vi "AD.vi"() -> ()   [LabVIEW 2018]
uses:
  work2020/SARController/SAR-Controller/main/PCI8552B_32.dll
panel:
  out "Data":dbl[][](array[numeric])
  out "波形图":dbl[][](graph)
  out "待读取数据长度":i32
  in  "STOP":bool
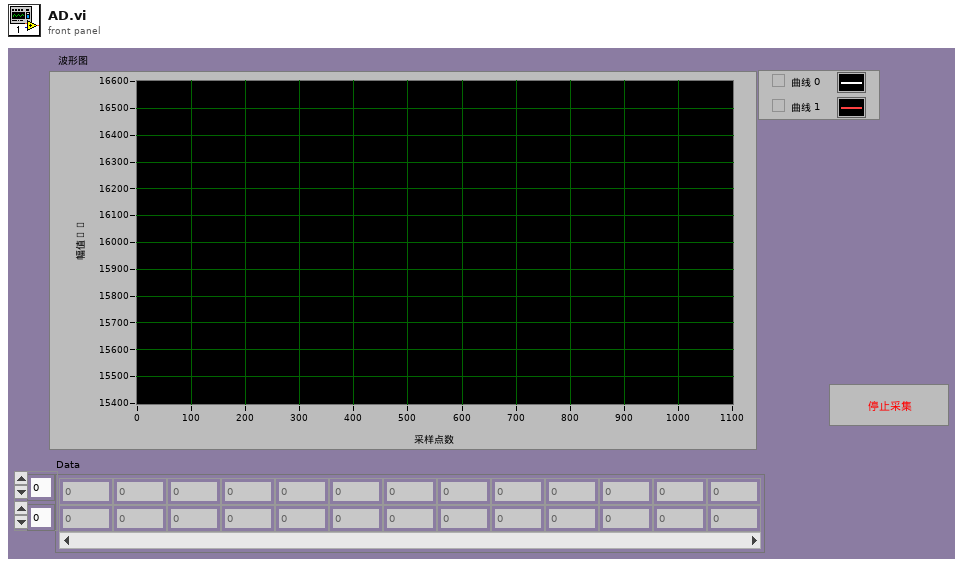
[diagram p1: front panel]
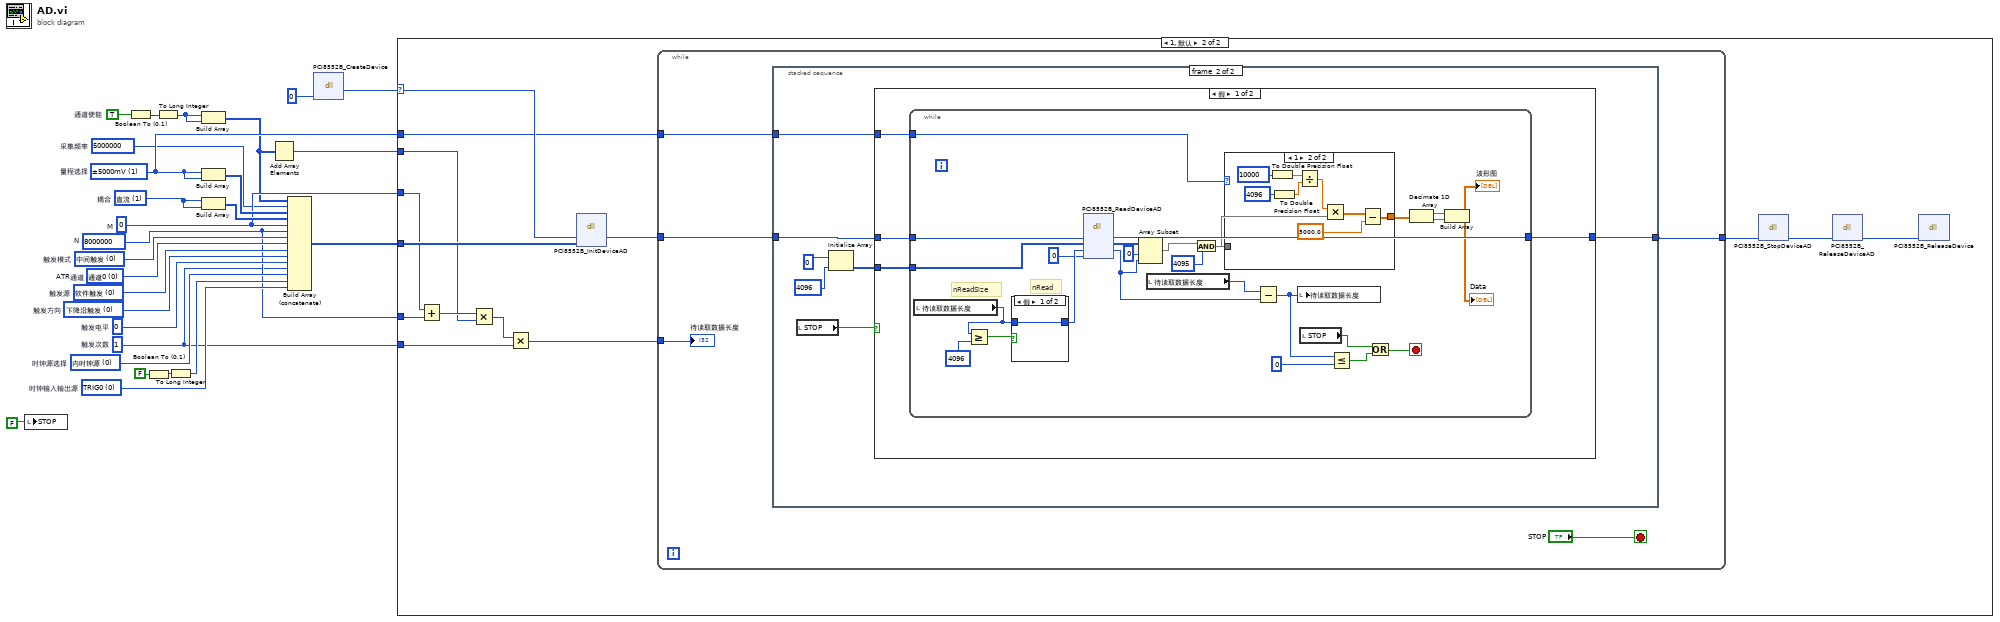
[diagram p0: block diagram]
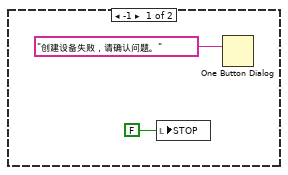
[diagram p2: hidden frame]
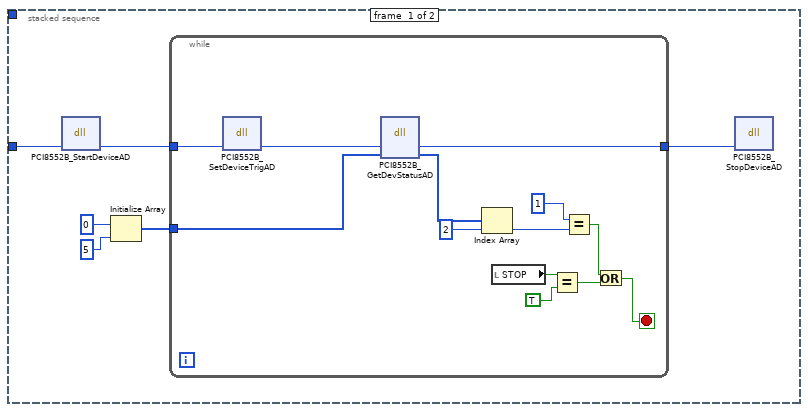
[diagram p3: hidden frame]
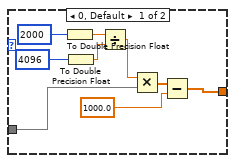
[diagram p4: hidden frame]
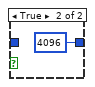
[diagram p5: hidden frame]
diagram:
  w6 = 8000000  # N
  w7 = 0  # M
  w8 = 1 items=["交流", "直流"]  # 耦合
  w3 = 1 items=["±1000mV", "±5000mV"]  # 量程选择
  w10 = TRUE  # 通道使能
  w1 = 5000000  # 采集频率
  w16 = 0 items=["中间触发", "后触发", "预触发", "硬件延时触发"]  # 触发模式
  w13 = 0 items=["通道0", "通道1"]  # ATR通道
  w25 = 0 items=["软件触发", "DTR作为触发源", "ATR作为触发源", "Trigger信号触发"]  # 触发源
  w24 = 0 items=["下降沿触发", "上升沿触发", "上下边沿均触发", ""]  # 触发方向
  w23 = 0  # 触发电平
  w4 = 1  # 触发次数
  w21 = 0 items=["TRIG0", "TRIG1", "TRIG2", "TRIG3"]  # 时钟输入输出源
  w22 = 0 items=["内时钟源", "主卡10M时钟源", "外部时钟"]  # 时钟源选择
  n1 = local write "STOP"(FALSE) -> ()
  n2 = Boolean To (0,1)(Boolean=w10) -> (0, 1=w18:i16)
  n3 = Boolean To (0,1)(Boolean=FALSE ("主设备使能")) -> (0, 1=w19:i16)
  n4 = To Long Integer(number=w18) -> (32bit integer=w9:i32)
  n5 = To Long Integer(number=w19) -> (32bit integer=w20:i32)
  n6 = Build Array(w9, w9) -> (w2:i32[])
  n7 = Build Array(w3, w3) -> (w15:i32[])
  n8 = Build Array(w8, w8) -> (w26:i32[])
  n9 = Add Array Elements(numeric array=w2) -> (sum=w5:i32)
  n10 = Build Array (concatenate)(w2, w1, w15, w26, w7, w6, w16, w13, w25, w24, w23, w4, w22, w20, w21) -> (w17:i32[])
  n11 = dll-call lib="PTH2…abs E\nPersonal Fileç ”ç©¶ç”Ÿå­¦ä¹ 202002-202007ç ”ä¸€ä¸‹å­¦æœŸwork2020\nSARControllerSAR-ControllermainPCI8552B_32.DLL" fn="PCI8552B_CreateDevice" label="CreateDevice"("DeviceLgcID"=0) -> ("返回类型"=w11:i32)  [unwired: 4 in, 2 out]
  n12 = case shown="1, 默认" w11 {
    selector: w11 -> [_ w31]
    tunnel: w17 -> [_ w41]
    tunnel: w7 -> [_ w40]
    tunnel: w6 -> [_ w39]
    tunnel: w5 -> [_ w37]
    tunnel: w4 -> [_ w35]
    tunnel: w3 -> [_ w30]
    frame -1 {
      n13 = local write "STOP"(FALSE) -> ()
      n14 = One Button Dialog(message="创建设备失败，请确认问题。") -> ()  [unwired: 1 in, 1 out]
    }
    frame 1, Default {
      n15 = Add(x=w40, y=w39) -> (x+y=w38:i32)
      n16 = Multiply(x=w38, y=w37) -> (x*y=w36:i32)
      n17 = Multiply(x=w36, y=w35) -> (x*y=w34:i32)
      n18 = dll-call lib="PTH2…abs E\nPersonal Fileç ”ç©¶ç”Ÿå­¦ä¹ 202002-202007ç ”ä¸€ä¸‹å­¦æœŸwork2020\nSARControllerSAR-ControllermainPCI8552B_32.DLL" fn="PCI8552B_InitDeviceAD" label="InitDeviceAD"("hDevice"=w31, "pADPara"=w41) -> ("hDevice"=w42:i32)  [unwired: 5 in, 2 out]
      n19 = while {
        tunnel: [w48] -> w43
        tunnel: w42 -> [w46]
        tunnel: w34 -> [w47]
        tunnel: w30 -> [w44]
        stop <- "STOP" stop-if-true
        n20 = stacked-sequence {
          tunnel: w46 -> [w50 w69]
          tunnel: [_ w74] -> w48
          tunnel: w44 -> [_ w68]
          frame #0 {
            n21 = dll-call lib="PTH2…abs E\nPersonal Fileç ”ç©¶ç”Ÿå­¦ä¹ 202002-202007ç ”ä¸€ä¸‹å­¦æœŸwork2020\nSARControllerSAR-ControllermainPCI8552B_32.DLL" fn="PCI8552B_StartDeviceAD" label="StartDeviceAD"("hDevice"=w50) -> ("hDevice"=w49:i32)  [unwired: 4 in, 2 out]
            n22 = Initialize Array(0, 5) -> (w54:i32[])
            n23 = while {
              tunnel: w49 -> [w57]
              tunnel: w54 -> [w67]
              tunnel: [w55] -> w51
              stop <- w58 stop-if-true
              n24 = dll-call lib="PTH2…abs E\nPersonal Fileç ”ç©¶ç”Ÿå­¦ä¹ 202002-202007ç ”ä¸€ä¸‹å­¦æœŸwork2020\nSARControllerSAR-ControllermainPCI8552B_32.DLL" fn="PCI8552B_SetDeviceTrigAD" label="SetDeviceTrigAD"("hDevice"=w57) -> ("hDevice"=w56:i32)  [unwired: 4 in, 2 out]
              n25 = dll-call lib="PTH2…abs E\nPersonal Fileç ”ç©¶ç”Ÿå­¦ä¹ 202002-202007ç ”ä¸€ä¸‹å­¦æœŸwork2020\nSARControllerSAR-ControllermainPCI8552B_32.DLL" fn="PCI8552B_GetDevStatusAD" label="GetDevStatusAD"("hDevice"=w56, "ADStatus"=w67) -> ("hDevice"=w55:i32, "ADStatus"=w63:i32[])  [unwired: 4 in, 2 out]
              n26 = Index Array(array=w63, index=2) -> (element=w65:i32)
              n27 = local read "STOP"() -> (w62:bool)
              n28 = Equal?(x=w62, y=TRUE) -> (x = y?=w59:bool)
              n29 = Equal?(x=1, y=w65) -> (x = y?=w60:bool)
              n30 = Or(x=w60, y=w59) -> (x .or. y?=w58:bool)
            }
            n31 = dll-call lib="PTH2…abs E\nPersonal Fileç ”ç©¶ç”Ÿå­¦ä¹ 202002-202007ç ”ä¸€ä¸‹å­¦æœŸwork2020\nSARControllerSAR-ControllermainPCI8552B_32.DLL" fn="PCI8552B_StopDeviceAD" label="StopDeviceAD"("hDevice"=w51) -> ()  [unwired: 5 in, 2 out]
          }
          frame #1 {
            n32 = local read "STOP"() -> (w70:bool)
            n33 = Initialize Array(u16 0 ("y"), 4096 ("y")) -> (w71:u16[])
            n34 = case shown="假" w70 {
              tunnel: w69 -> [w78 w124]
              tunnel: [w77 w124] -> w74
              tunnel: w71 -> [w76 _]
              tunnel: w68 -> [w75 _]
              frame False {
                n35 = while {
                  tunnel: w78 -> [w103]
                  tunnel: [w102] -> w77
                  tunnel: w76 -> [w101]
                  tunnel: w75 -> [w88]
                  stop <- w96 stop-if-true
                  # "nReadSize"
                  # "nRead"
                  n36 = local read "待读取数据长度"() -> (w95:i32)
                  n37 = Greater Or Equal?(x=w95, y=4096 ("millisecond multiple")) -> (x >= y?=w99:bool)
                  n38 = case shown="假" w99 {
                    tunnel: [w122 4096 ("millisecond multiple")] -> w92
                    tunnel: w95 -> [w122 _]
                    frame False {
                    }
                    frame True {
                    }
                  }
                  n39 = dll-call lib="PTH2…abs E\nPersonal Fileç ”ç©¶ç”Ÿå­¦ä¹ 202002-202007ç ”ä¸€ä¸‹å­¦æœŸwork2020\nSARControllerSAR-ControllermainPCI8552B_32.DLL" fn="PCI8552B_ReadDeviceAD" label="ReadDeviceAD"("hDevice"=w103, "pADBuffer"=w101, "nReadSizeWords"=w92, "nRetSizeWords"=0) -> ("hDevice"=w102:i32, "pADBuffer"=w85:u16[], "nReadSizeWords"=w82:u32)  [unwired: 5 in, 2 out]
                  n40 = Array Subset(array=w85, index=0 ("索引"), length=w82) -> (w84:u16[])
                  n41 = local read "待读取数据长度"() -> (w94:i32)
                  n42 = And(x=w84, y=u16 4095) -> (x .and. y?=w89:u16[])
                  n43 = case shown="1" w88 {
                    tunnel: w89 -> [w111 w116]
                    tunnel: [w104 w115] -> w87
                    frame 0, Default {
                      n44 = To Double Precision Float(number=2000 ("x")) -> (double precision float=w107:dbl)
                      n45 = To Double Precision Float(number=4096) -> (double precision float=w106:dbl)
                      n46 = Divide(x=w107, y=w106) -> (x/y=w112:dbl)
                      n47 = Multiply(x=w112, y=w111) -> (x*y=w110:dbl[])
                      n48 = Subtract(x=w110, y=1000.0) -> (x-y=w104:dbl[])
                    }
                    frame 1 {
                      n49 = To Double Precision Float(number=10000 ("x")) -> (double precision float=w114:dbl)
                      n50 = To Double Precision Float(number=4096) -> (double precision float=w118:dbl)
                      n51 = Divide(x=w114, y=w118) -> (x/y=w121:dbl)
                      n52 = Multiply(x=w121, y=w116) -> (x*y=w120:dbl[])
                      n53 = Subtract(x=w120, y=5000.0) -> (x-y=w115:dbl[])
                    }
                  }
                  n54 = Subtract(x=w94, y=w82) -> (x-y=w93:u32)
                  n55 = local write "待读取数据长度"(w93) -> ()
                  n56 = local read "STOP"() -> (w91:bool)
                  n57 = Less Or Equal?(x=w93, y=0) -> (x <= y?=w97:bool)
                  n58 = Or(x=w91, y=w97) -> (x .or. y?=w96:bool)
                  n59 = Decimate 1D Array(w87) -> (w81:dbl[], w80:dbl[])
                  n60 = Build Array(w81, w80) -> (→"波形图" →"Data":dbl[][])
                }
              }
              frame True {
              }
            }
          }
        }
        "待读取数据长度" <- w47
      }
      n61 = dll-call lib="PTH2…abs E\nPersonal Fileç ”ç©¶ç”Ÿå­¦ä¹ 202002-202007ç ”ä¸€ä¸‹å­¦æœŸwork2020\nSARControllerSAR-ControllermainPCI8552B_32.DLL" fn="PCI8552B_StopDeviceAD" label="StopDeviceAD"("hDevice"=w43) -> ("hDevice"=w33:i32)  [unwired: 4 in, 2 out]
      n62 = dll-call lib="PTH2…abs E\nPersonal Fileç ”ç©¶ç”Ÿå­¦ä¹ 202002-202007ç ”ä¸€ä¸‹å­¦æœŸwork2020\nSARControllerSAR-ControllermainPCI8552B_32.DLL" fn="PCI8552B_ReleaseDeviceAD" label="ReleaseDeviceAD"("hDevice"=w33) -> ("hDevice"=w32:i32)  [unwired: 4 in, 2 out]
      n63 = dll-call lib="PTH2…abs E\nPersonal Fileç ”ç©¶ç”Ÿå­¦ä¹ 202002-202007ç ”ä¸€ä¸‹å­¦æœŸwork2020\nSARControllerSAR-ControllermainPCI8552B_32.DLL" fn="PCI8552B_ReleaseDevice" label="ReleaseDevice"("hDevice"=w32) -> ()  [unwired: 5 in, 2 out]
    }
  }
